vi "Enforce Robot Rules.vi"(5 "max V":dbl, 6 "Arr Refnum":refnum<vi>, 7 "Clust Refnum":refnum<vi>, 9 "Disable":bool, 10 "New Points":cluster{"x":dbl, "y":dbl, "th":dbl}[](array[cluster]), 11 "Original Points":cluster{"x":dbl, "y":dbl, "th":dbl}[](array[cluster])) -> (3 "Points out":cluster{"x":dbl, "y":dbl, "th":dbl}[](array[cluster]))   [LabVIEW 2019]
panel:
  # "1"
  # "2"
  # "3"
  # "4"
  # "5"
  # "6"
  # "7"
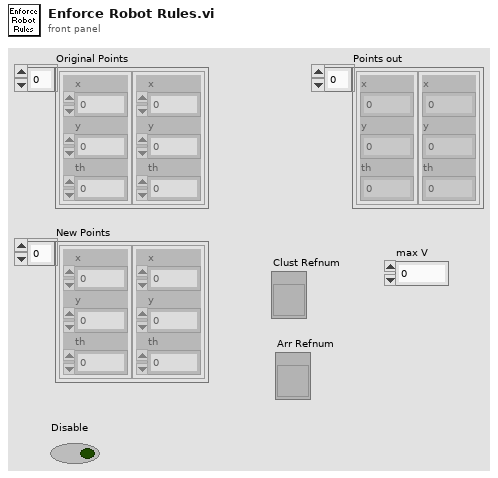
[diagram p1: front panel]
types:
  T1 = cluster{"Angular \nAccelerations":dbl[], "Override Limits?":bool[]}
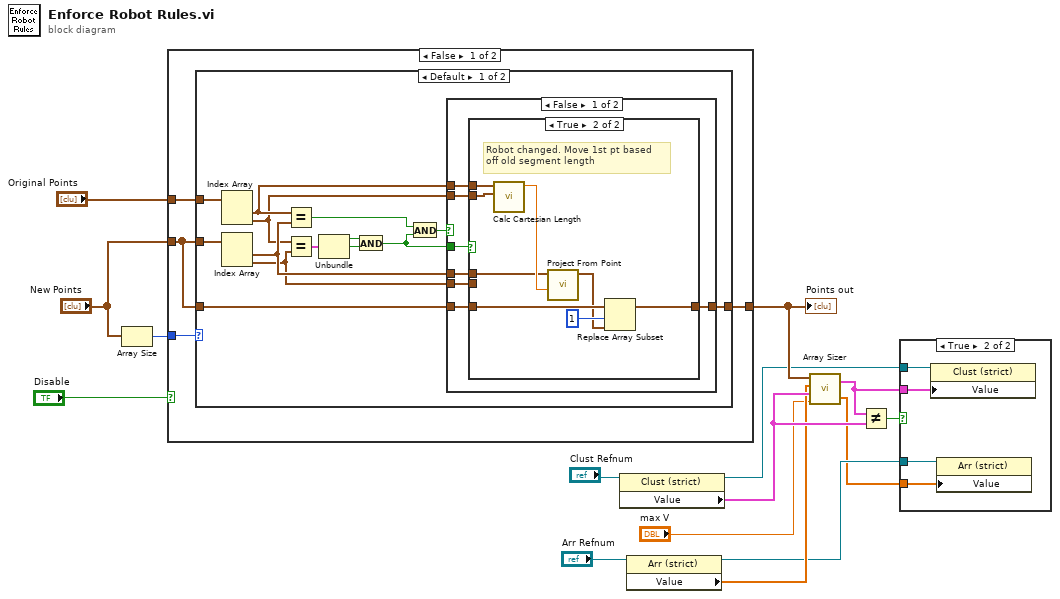
[diagram p0: block diagram]
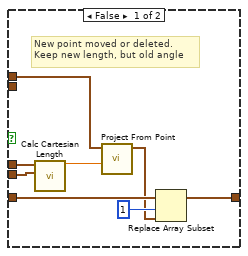
[diagram p3: hidden frame]
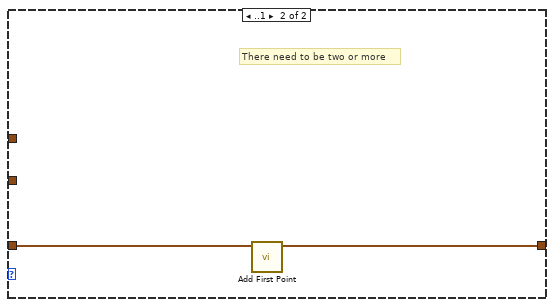
[diagram p5: hidden frame]
diagram:
  n1 = Array Size(array="New Points") -> (size(s)=w14:i32)
  n2 = case shown="False" "Disable" {
    tunnel: "Original Points" -> [w19 _]
    tunnel: w14 -> [w18 _]
    tunnel: [w17 w60] -> w11
    tunnel: "New Points" -> [w16 w60]
    frame False {
      n3 = case shown="Default" w18 {
        tunnel: w19 -> [w33 _]
        tunnel: w16 -> [w32 _]
        tunnel: [w30 w59] -> w17
        tunnel: w16 -> [w29 w58]
        frame Default {
          n4 = Index Array(array=w33) -> (element #1=w27:cluster{"x":dbl, "y":dbl, "th":dbl}, element #2=w24:cluster{"x":dbl, "y":dbl, "th":dbl})  [unwired: 2 in]
          n5 = Index Array(array=w32) -> (element #1=w26:cluster{"x":dbl, "y":dbl, "th":dbl}, element #2=w25:cluster{"x":dbl, "y":dbl, "th":dbl})  [unwired: 2 in]
          n6 = Equal?(x=w27, y=w26) -> (x = y?=w28:bool)
          n7 = Equal?(x=w24, y=w25) -> (x = y?=w23:cluster{"x":bool, "y":bool, "th":bool})
          n8 = Unbundle(w23) -> ("x"=w22:bool, "y"=w21:bool)  [unwired: 1 out]
          n9 = And(x=w22, y=w21) -> (x .and. y?=w20:bool)
          n10 = And(x=w28, y=w20) -> (x .and. y?=w31:bool)
          n11 = case shown="False" w31 {
            tunnel: [w36 w57] -> w30
            tunnel: w29 -> [w34 w57]
            tunnel: w20 -> [w38 _]
            tunnel: w27 -> [w40 _]
            tunnel: w24 -> [w39 _]
            tunnel: w26 -> [w37 _]
            tunnel: w25 -> [w35 _]
            frame False {
              n12 = case shown="True" w38 {
                tunnel: w40 -> [w43 w56]
                tunnel: w39 -> [_ w55]
                tunnel: w37 -> [w48 w50]
                tunnel: [w44 w53] -> w36
                tunnel: w35 -> [w47 _]
                tunnel: w34 -> [w45 w54]
                frame False {
                  # "New point moved or deleted.\nKeep new length, but old angle"
                  n13 = call "Calc Cartesian Length.vi"("Point 2"=w47, "Point 1"=w48) -> ("Length (f)"=w42:dbl)  [unwired: 8 in, 1 out]
                  n14 = call "Project From Point.vi"("distance"=w42, "Point In"=w43) -> ("Point Out"=w41:cluster{"x":dbl, "y":dbl, "th":dbl})  [unwired: 9 in]
                  n15 = Replace Array Subset(array=w45, new element=w41, index=1) -> (w44:cluster{"x":dbl, "y":dbl, "th":dbl}[])
                }
                frame True {
                  # "Robot changed. Move 1st pt based\noff old segment length"
                  n16 = call "Calc Cartesian Length.vi"("Point 2"=w55, "Point 1"=w56) -> ("Length (f)"=w51:dbl)  [unwired: 8 in, 1 out]
                  n17 = call "Project From Point.vi"("distance"=w51, "Point In"=w50) -> ("Point Out"=w49:cluster{"x":dbl, "y":dbl, "th":dbl})  [unwired: 9 in]
                  n18 = Replace Array Subset(array=w54, new element=w49, index=1) -> (w53:cluster{"x":dbl, "y":dbl, "th":dbl}[])
                }
              }
            }
            frame True {
              # "First two elements didn't\nchange. assume they are\ngood"
            }
          }
        }
        frame ..1 {
          # "There need to be two or more"
          n19 = call "Add First Point.vi"("Initial Points"=w58) -> ("Points"=w59:cluster{"x":dbl, "y":dbl, "th":dbl}[])  [unwired: 10 in]
        }
      }
    }
    frame True {
    }
  }
  "Points out" <- w11
  n20 = property class="Clust (strict)"(reference="Clust Refnum") -> (reference out=w9:refnum<vi>, "Value"=w7:T1)  [unwired: 1 in, 1 out]
  n21 = property class="Arr (strict)"(reference="Arr Refnum") -> (reference out=w3:refnum<vi>, "Value"=w4:dbl[])  [unwired: 1 in, 1 out]
  n22 = call "Array Sizer.vi"("maxV"="max V", "Angular Accelerations"=w7, "Velocities"=w4, "Points out"=w11) -> ("Velocities out"=w2:dbl[], "output cluster"=w8:T1)
  n23 = Not Equal?(x=w8, y=w7) -> (x != y?=w6:bool)
  n24 = case shown="True" w6 {
    tunnel: w8 -> [_ w64]
    tunnel: w9 -> [_ w63]
    tunnel: w3 -> [_ w62]
    tunnel: w2 -> [_ w61]
    frame False {
    }
    frame True {
      n25 = property class="Clust (strict)"(reference=w63, "Value"=w64) -> ()  [unwired: 1 in, 2 out]
      n26 = property class="Arr (strict)"(reference=w62, "Value"=w61) -> ()  [unwired: 1 in, 2 out]
    }
  }
